vi "Start Communication 9620.vi"(8 "error in":errorcluster, 11 "VISA resource name":refnum<visa-resource-name>="COM3") -> (0 "error out":errorcluster, 3 "VISA out":refnum<visa-resource-name>)   [LabVIEW 2017]
doc: "This example performs writes and reads on a serial port, as directed by the user. You can press the Write and Read buttons, and change the Read Count, while the example is running.\n\nThe parameters set for the serial port must match the parameters of the connected instrument or device. In this example, the Read Count parameter specifies the number of bytes that the serial port reads. If there were more bytes at the port than the specified number, those bytes would not be read. If there were less bytes at the port than the specified number, you would receive a timeout error.\n\nThis example expands upon the flow control options for XON and XOFF, allowing the user to choose those control characters. Also, the user can enable or disable a termination character. Some devices require a termination character in order to identify the end of command strings. Some devices send a termination character to signify the end of data to be read. This example shows how you can end the Read operation once a termination character is detected in the buffer and/or append a termination character at the end of the Write data."
uses:
  <vilib>/Instr/_visa.llb/VISA Configure Serial Port (Instr).vi
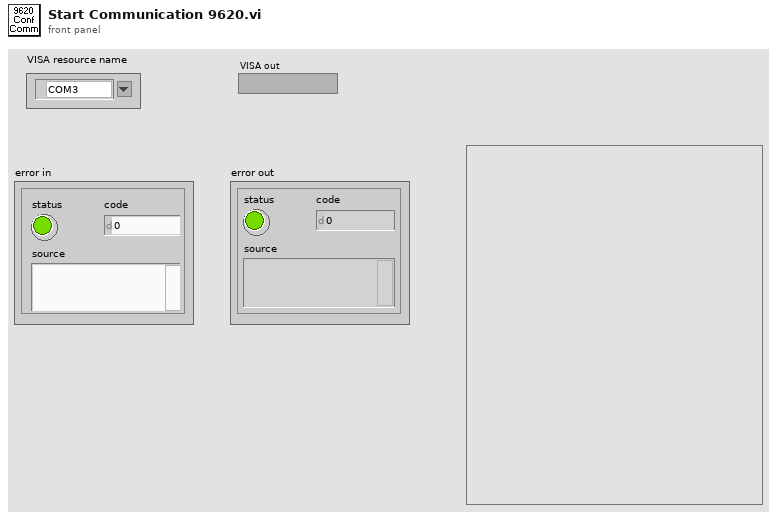
[diagram p1: front panel]
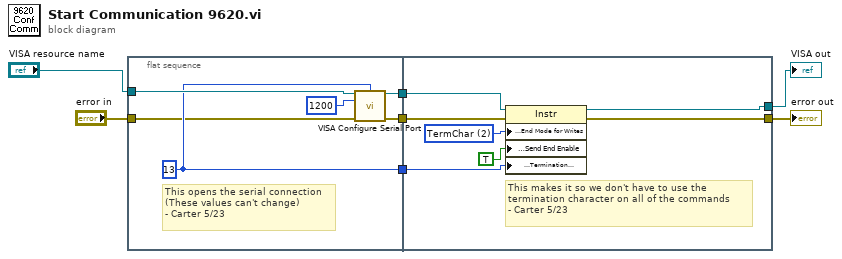
[diagram p0: block diagram]
diagram:
  n1 = flat-sequence {
    tunnel: "VISA resource name" -> [w13]
    tunnel: "error in" -> [w8]
    tunnel: [w12] -> w5
    tunnel: [w11] -> w4
    tunnel: [w10] -> w3
    tunnel: w5 -> [w20]
    tunnel: w4 -> [w19]
    tunnel: w3 -> [w16]
    tunnel: [w15] -> w2
    tunnel: [w14] -> w1
    frame #0 {
      w10 = u8 13 ("Termination Character")
      # "This opens the serial connection\n(These values can't change)\n- Carter 5/23"
      n2 = call-poly "VISA Configure Serial Port"("VISA resource name"=w13, "termination char\n(0xA = '\\n' = LF)"=w10, "baud rate (9600)"=u32 1200, "error in (no error)"=w8) -> ("VISA resource name out"=w12:refnum<visa-resource-name>, "error out"=w11:errorcluster)  [unwired: 6 in, 4 out]
    }
    frame #1 {
      w18 = u16 2 items=["None", "LastBit", "TermChar", "Break"] ("Serial Settings:Serial End Mode for Writes")
      # "This makes it so we don't have to use the \ntermination character on all of the commands\n- Carter 5/23"
      n3 = property class="Instr"(reference=w20, error in=w19, "Serial Settings:End Mode for Writes"=w18, "Message Based Settings:Send End Enable"=TRUE, "Message Based Settings:Termination Character"=w16) -> (reference out=w15:refnum<visa-resource-name>, error out=w14:errorcluster)
    }
  }
  "VISA out" <- w2
  "error out" <- w1
